vi "configureAcquisition.vi"(6 "imagePaths":path[](array[path]), 7 "saveImages?":bool, 8 "error in (no error)":errorcluster, 9 "number of Images":i32, 10 "CameraSettings":refnum<class "CamaraSettings.lvclass">, 11 "ProEM_WinX32 in":refnum<class "ProEM_WinX32.lvclass">) -> (0 "error out":errorcluster, 3 "ProEM_WinX32 out":refnum<class "ProEM_WinX32.lvclass">)   [LabVIEW 2009, in "Hardware.lvlib" / "Channels.lvlib" / "ProEM_WinX32.lvclass"]
doc: "Camera Settings are made from within WinX32 software.\nThey are not changed here.\nOnly the total number of images to take in the acquisition is set from here"
uses:
  ProEM_WinX32.lvclass
  Tools/CameraSettings/CamaraSettings.lvclass
  Camera/Camera.lvclass
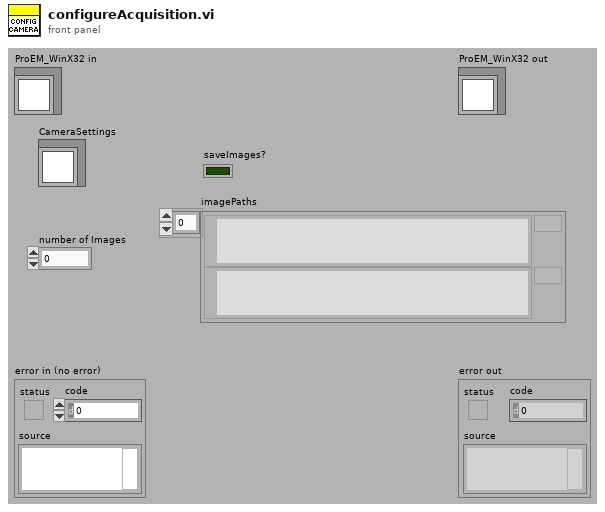
[diagram p1: front panel]
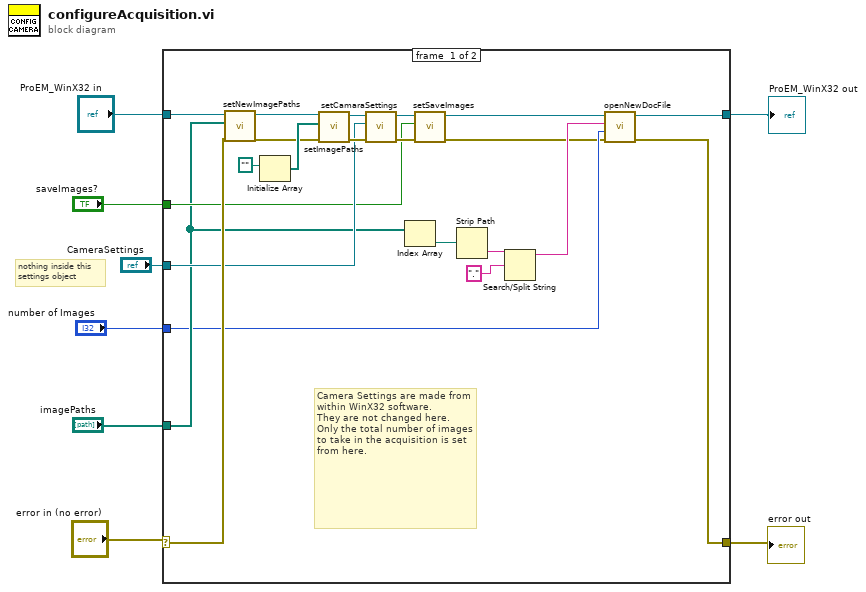
[diagram p0: block diagram]
diagram:
  # "nothing inside this\nsettings object"
  n1 = case shown="No Error" "error in (no error)" {
    selector: "error in (no error)" -> [w29 w31]
    tunnel: [w12 w32] -> w8
    tunnel: "ProEM_WinX32 in" -> [w30 w32]
    tunnel: [w11 w31] -> w5
    tunnel: "saveImages?" -> [w19 _]
    tunnel: "CameraSettings" -> [w22 _]
    tunnel: "number of Images" -> [w13 _]
    tunnel: "imagePaths" -> [w18 _]
    frame #0 {
      # "Camera Settings are made from within WinX32 software.\nThey are not changed here.\nOnly the total number of images to take in the acquisition is set from here."
      n2 = call "setNewImagePaths.vi"("error in (no error)"=w29, "NewImagePaths"=w18, "Camera in"=w30) -> ("error out"=w26:errorcluster, "Camera out"=w25:refnum<class "ProEM_WinX32.lvclass">)  [unwired: 7 in]
      n3 = Initialize Array(path "") -> (w27:path[])  [unwired: 1 in]
      n4 = call "setImagePaths.vi"("error in (no error)"=w26, "ImagePaths"=w27, "Camera in"=w25) -> ("error out"=w23:errorcluster, "Camera out"=w24:refnum<class "ProEM_WinX32.lvclass">)  [unwired: 7 in]
      n5 = call "setCamaraSettings.vi"("error in (no error)"=w23, "CamaraSettings"=w22, "Camera in"=w24) -> ("error out"=w20:errorcluster, "Camera out"=w21:refnum<class "ProEM_WinX32.lvclass">)  [unwired: 7 in]
      n6 = Index Array(array=w18) -> (element=w17:path)  [unwired: 1 in]
      n7 = call "setSaveImages.vi"("error in (no error)"=w20, "saveImages?"=w19, "Camera in"=w21) -> ("error out"=w9:errorcluster, "Camera out"=w10:refnum<class "ProEM_WinX32.lvclass">)  [unwired: 7 in]
      n8 = Strip Path(path=w17) -> (name=w16:string)  [unwired: 1 out]
      n9 = Search/Split String(string=w16, search string/char (-)=".") -> (substring before match=w14:string)  [unwired: 1 in, 2 out]
      n10 = call "openNewDocFile.vi"("error in (no error)"=w9, "# of images"=w13, "name"=w14, "ProEM_WinX32 in"=w10) -> ("error out"=w11:errorcluster, "ProEM_WinX32 out"=w12:refnum<class "ProEM_WinX32.lvclass">)  [unwired: 6 in]
    }
    frame #1 {
    }
  }
  "error out" <- w5
  "ProEM_WinX32 out" <- w8
